vi "Get SMO PGSQL Log Paths.vi"(5 "getAll Cluster":variant, 7 "Default Paths":string, 8 "error in (no error)":errorcluster, 11 "Example in":refnum<class "Instrument.Element2.lvclass">) -> (0 "error out":errorcluster, 2 "Paths":string, 3 "Example out":refnum<class "Instrument.Element2.lvclass">)   [LabVIEW 2019, in "Instrument.Element2.lvclass"]
uses:
  Instrument.Element2.lvclass
  <userlib>/LevyLab/Instrument Framework/Instrument Types/VSource/Instrument.VSource.lvclass
  Typedefs/Instrument.Element2.getAll--Cluster.ctl
  <userlib>/LevyLab/LV-Data/LV-Data.PG/LV-Data.PGSQL.lvclass
  <userlib>/LevyLab/LV-Data/LV-Data.PG/API/Write Variable (one-row).vi
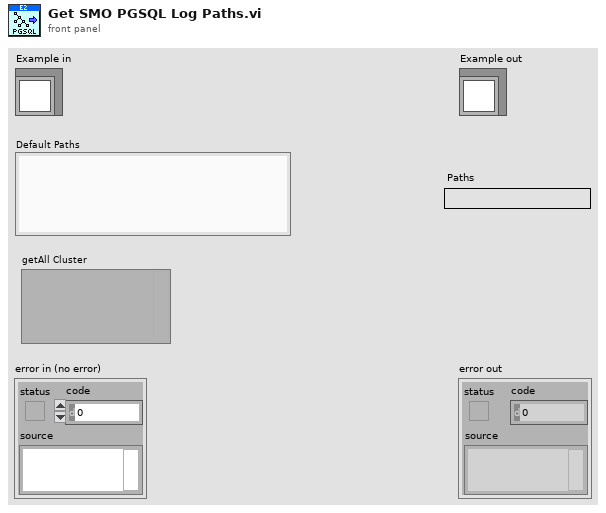
[diagram p1: front panel]
types:
  T1 = typedef "Instrument.Element2.lvclass/Instrument.Element2.getAll--Cluster.ctl" = cluster{"Pump Power":dbl, "Laser Status":string, "Startup/Shutdown Status":string, "Diode Current Set":dbl, "Diode Current Actual":dbl, "Temp: Pump Chassis":dbl, "Temp: Pump PCB":dbl, "Temp: Pump Tower":dbl, "Temp: Pump Diodes":dbl, "Temp: Control Unit":dbl, "Temp: Laser Head Pos 1":dbl, "Temp: Laser Head Pos 2":dbl}
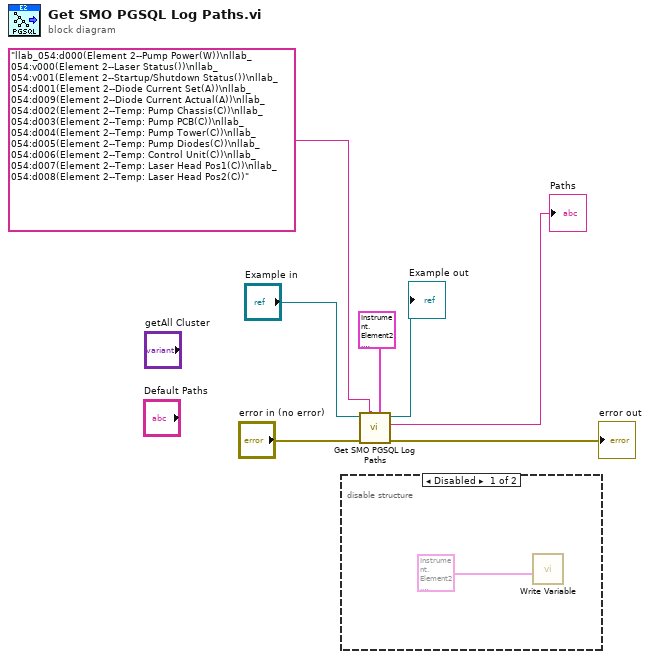
[diagram p0: block diagram]
diagram:
  n1 = disable-structure shown="Disabled" {
    frame Disabled {
      n2 = call-poly <userlib>:"Write Variable.vi"("Data"=T1 {"Pump Power"=0.0, "Laser Status"="", "Startup/Shutdown Status"="", "Diode Current Set"=0.0, "Diode Current Actual"=0.0, "Temp: Pump Chassis"=0.0, "Temp: Pump PCB"=0.0, "Temp: Pump Tower"=0.0, "Temp: Pump Diodes"=0.0, "Temp: Control Unit"=0.0, "Temp: Laser Head Pos 1"=0.0, "Temp: Laser Head Pos 2"=0.0} ("getAll")) -> ()  [unwired: 7 in, 4 out]
    }
    frame Enabled {
    }
  }
  n3 = call-parent "Get SMO PGSQL Log Paths.vi"("getAll Cluster"=T1 {"Pump Power"=0.0, "Laser Status"="", "Startup/Shutdown Status"="", "Diode Current Set"=0.0, "Diode Current Actual"=0.0, "Temp: Pump Chassis"=0.0, "Temp: Pump PCB"=0.0, "Temp: Pump Tower"=0.0, "Temp: Pump Diodes"=0.0, "Temp: Control Unit"=0.0, "Temp: Laser Head Pos 1"=0.0, "Temp: Laser Head Pos 2"=0.0} ("getAll"), "Default Paths"="llab_054:d000(Element 2--Pump Power(W))\nllab_054:v000(Element 2--Laser Status())\nllab_054:v001(Element 2--Startup/Shutdown Status())\nllab_054:d001(Element 2--Diode Current Set(A))\nllab_054:d009(Element 2--Diode Current Actual(A))\nllab_054:d002(Element 2--Temp: Pump Chassis(C))\nllab_054:d003(Element 2--Temp: Pump PCB(C))\nllab_054:d004(Element 2--Temp: Pump Tower(C))\nllab_054:d005(Element 2--Temp: Pump Diodes(C))\nllab_054:d006(Element 2--Temp: Control Unit(C))\nllab_054:d007(Element 2--Temp: Laser Head Pos1(C))\nllab_054:d008(Element 2--Temp: Laser Head Pos2(C))" ("Paths"), "error in (no error)"="error in (no error)", "Instrument in"="Example in") -> ("error out"=→"error out":errorcluster, "Paths"=→"Paths":string, "Instrument out"=→"Example out":refnum<class "Instrument.Element2.lvclass">)  [unwired: 5 in]
